vi "tearDown.vi"(8 "error in (no error)":errorcluster, 11 "TestConfigurationFileBinding In":refnum<class "TestConfigurationFileBinding.lvclass">) -> (0 "error out":errorcluster, 3 "TestConfigurationFileBinding Out":refnum<class "TestConfigurationFileBinding.lvclass">)   [LabVIEW 2017, in "TestConfigurationFileBinding.lvclass"]
doc: "tearDown runs after the test method has completed. Use this method to clean up any operations or references that were opened by setUp or the test method. Unit tests should be independent of other unit tests so this VI should ensure that the next test can run in a 'clean' test environment."
uses:
  TestConfigurationFileBinding.lvclass
  TestConfigurationFileBinding.lvclass/TestConfigurationFileBinding.ctl
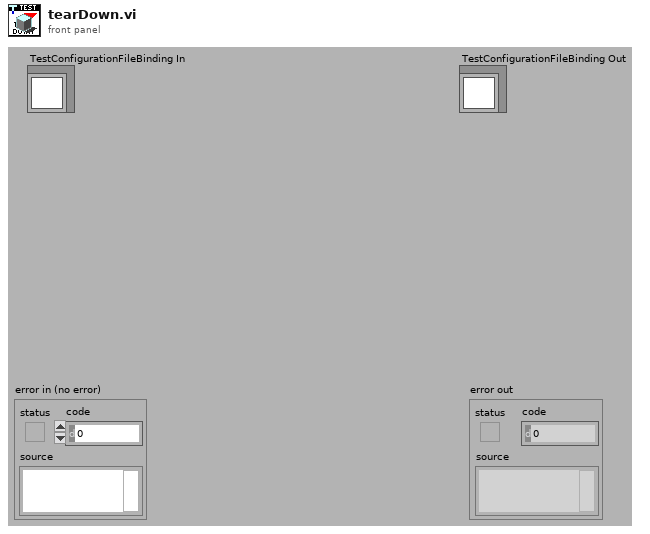
[diagram p1: front panel]
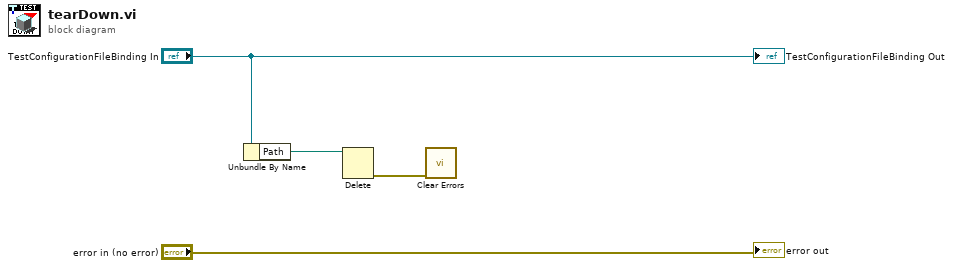
[diagram p0: block diagram]
diagram:
  n1 = Unbundle By Name("TestConfigurationFileBinding In") -> ("Path"=w2:path)
  n2 = Delete(path (use dialog)=w2) -> (error out=w1:errorcluster)  [unwired: 4 in, 2 out]
  n3 = call <vilib>:"Clear Errors.vi"("error in (no error)"=w1) -> ()  [unwired: 5 in, 2 out]
  "error out" <- "error in (no error)"
  "TestConfigurationFileBinding Out" <- "TestConfigurationFileBinding In"
